vi "Tag.Properties.vi"(7 "Action":enum8{"Get", "Set"}(ring), 8 "error in (no error)":errorcluster, 10 "Channel Settings":T1, 11 "Section Ref in":T2 format="%.0x") -> (0 "error out":errorcluster, 2 "Channel Settings":T1, 3 "Item Ref out":T2 format="%.0x")   [LabVIEW 2015, in "OPC UA Client System Explorer.lvlib"]
uses:
  OPC UA Client System Explorer.lvlib
  <vilib>/NI Veristand/Custom Device API/Custom Device Item Ref.ctl
  Shared/Tag.Settings.ctl
  <vilib>/NI Veristand/Custom Device API/Get Item Property (U32).vi
  <vilib>/NI Veristand/Custom Device API/Get Item Property (String).vi
  <vilib>/NI Veristand/Custom Device API/Set Item Property (U32).vi
  <vilib>/NI Veristand/Custom Device API/Set Item Property (String).vi
  Shared/Constants.vi
  Shared/OPC UA Client Shared.lvlib
  <vilib>/NI VeriStand/Custom Device API/Custom Device API.lvlib
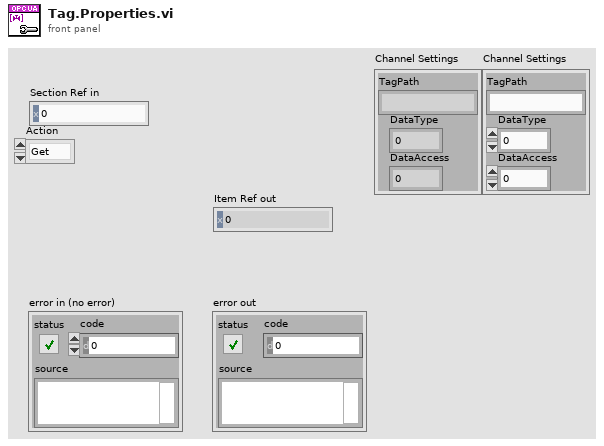
[diagram p1: front panel]
types:
  T1 = typedef "OPC UA Client Shared.lvlib/Tag.Settings.ctl" = cluster{"TagPath":string, "DataType":u32, "DataAccess":u32}
  T2 = typedef "Custom Device API.lvlib/Custom Device Item Ref.ctl" = u64
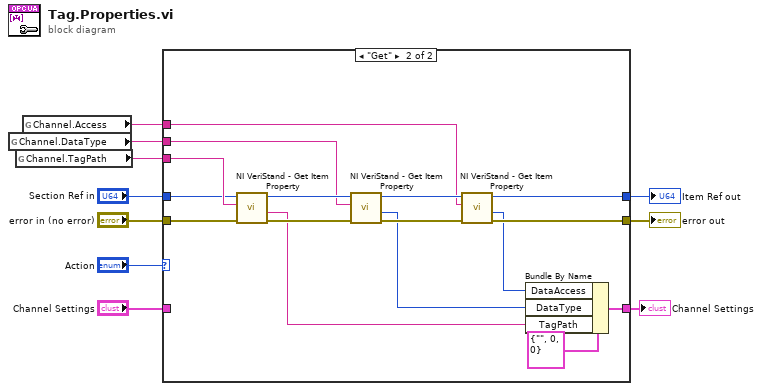
[diagram p0: block diagram]
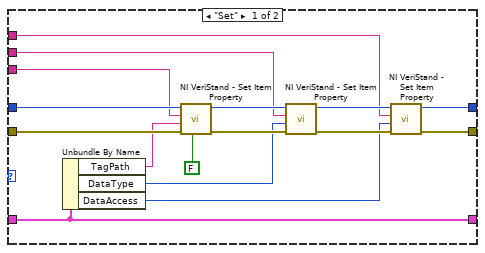
[diagram p2: hidden frame]
diagram:
  n1 = global read "Constants.vi" "Channel.DataType"() -> (w10:string)
  n2 = global read "Constants.vi" "Channel.TagPath"() -> (w7:string)
  n3 = global read "Constants.vi" "Channel.Access"() -> (w4:string)
  n4 = case shown="\"Get\"" "Action" {
    tunnel: w10 -> [w16 w38]
    tunnel: [w21 w37] -> w9
    tunnel: [w22 w36] -> w8
    tunnel: w7 -> [w17 w35]
    tunnel: "error in (no error)" -> [w26 w34]
    tunnel: "Section Ref in" -> [w18 w33]
    tunnel: w4 -> [w15 w31]
    tunnel: [w14 w27] -> w3
    tunnel: "Channel Settings" -> [w14 _]
    frame "Set" {
      n5 = Unbundle By Name(w14) -> ("TagPath"=w13:string, "DataType"=w12:u32, "DataAccess"=w11:u32)
      n6 = call-poly <vilib>:"NI VeriStand - Set Item Property.vi"("Binary String (T)"=FALSE, "error in (no error)"=w26, "Value"=w13, "Property Name"=w17, "Item Ref in"=w18) -> ("error out"=w24:errorcluster, "Item Ref out"=w19:T2)  [unwired: 4 in, 1 out]
      n7 = call-poly <vilib>:"NI VeriStand - Set Item Property.vi"("error in (no error)"=w24, "Value"=w12, "Property Name"=w16, "Item Ref in"=w19) -> ("error out"=w23:errorcluster, "Item Ref out"=w20:T2)  [unwired: 5 in, 1 out]
      n8 = call-poly <vilib>:"NI VeriStand - Set Item Property.vi"("error in (no error)"=w23, "Value"=w11, "Property Name"=w15, "Item Ref in"=w20) -> ("error out"=w22:errorcluster, "Item Ref out"=w21:T2)  [unwired: 5 in, 1 out]
    }
    frame "Get" {
      n9 = call-poly <vilib>:"NI VeriStand - Get Item Property.vi"("error in (no error)"=w34, "Property Name"=w35, "Item Ref in"=w33) -> ("error out"=w41:errorcluster, "Value"=w32:string, "Item Ref out"=w39:T2)  [unwired: 5 in, 1 out]
      n10 = call-poly <vilib>:"NI VeriStand - Get Item Property.vi"("error in (no error)"=w41, "Property Name"=w38, "Item Ref in"=w39) -> ("error out"=w42:errorcluster, "Value"=w28:u32, "Item Ref out"=w40:T2)  [unwired: 5 in, 1 out]
      n11 = call-poly <vilib>:"NI VeriStand - Get Item Property.vi"("error in (no error)"=w42, "Property Name"=w31, "Item Ref in"=w40) -> ("error out"=w36:errorcluster, "Value"=w29:u32, "Item Ref out"=w37:T2)  [unwired: 5 in, 1 out]
      n12 = Bundle By Name(cluster=T1 {"TagPath"="", "DataType"=0, "DataAccess"=0}, "DataAccess"=w29, "DataType"=w28, "TagPath"=w32) -> (w27:T1)
    }
  }
  "Item Ref out" <- w9
  "error out" <- w8
  "Channel Settings" <- w3
